vi "FITS read header.vi"() -> ()   [LabVIEW 2020]
panel:
  out "error out":errorcluster
  in  "error in":errorcluster
  out "Header":string[](array[string])
  out "data":string
  in  "Path":path
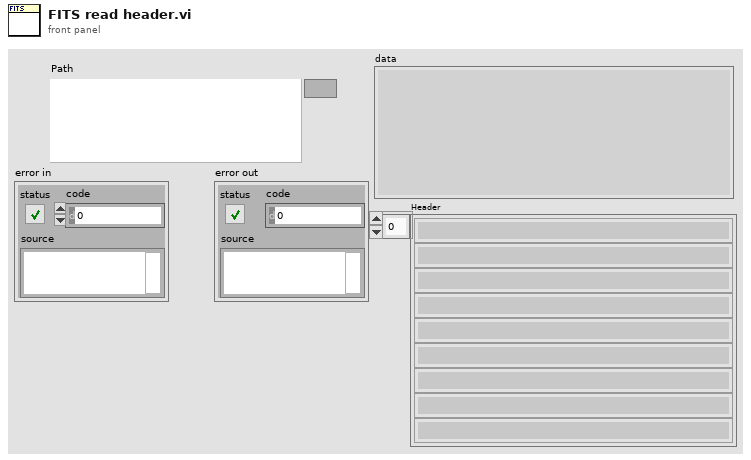
[diagram p1: front panel]
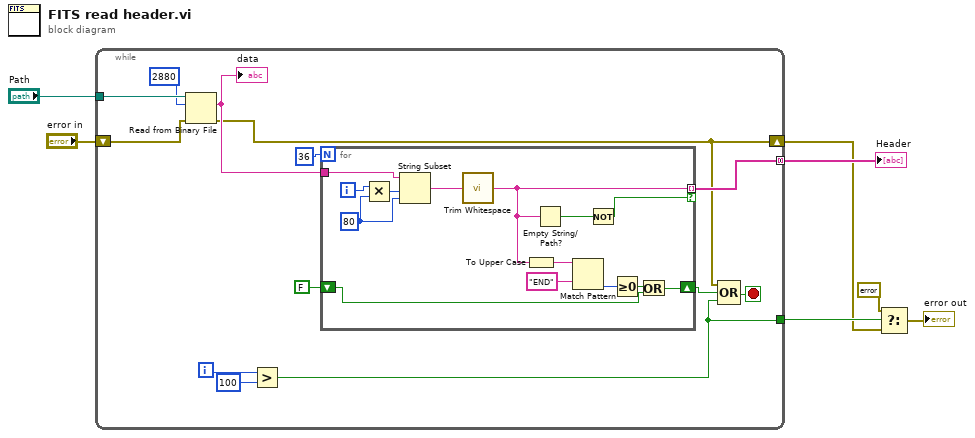
[diagram p0: block diagram]
diagram:
  n1 = while {
    tunnel: "Path" -> [w20]
    tunnel: [w16] -> w6 mode=concatenating
    tunnel: [w10] -> w4
    shift-right: [w8] -> w3
    shift-left: "error in" -> [w9]
    i -> [w13]
    stop <- w11 stop-if-true
    n2 = Read from Binary File(8:w9, 10:2880 ("count (1)"), 11:w20) -> (0:w8:errorcluster, 2:w18:string)  [unwired: 3 in, 2 out]
    "data" <- w18
    n3 = Greater?(x=w13, y=100) -> (0:w10:bool)
    n4 = for {
      N: 36 -> [_]
      tunnel: w18 -> [w34]
      tunnel: [w27] -> w16 mode=indexing if=w28
      shift-right: [w22] -> w14
      shift-left: FALSE -> [w21]
      i -> [w32]
      w31 = 80 ("length (rest)")
      n5 = Multiply(x=w32, y=w31) -> (x*y=w33:i32)
      n6 = String Subset(string=w34, offset (0)=w33, length (rest)=w31) -> (substring=w30:string)
      n7 = call <vilib>:"Trim Whitespace.vi"("string"=w30) -> ("trimmed string"=w27:string)  [unwired: 1 in]
      n8 = To Upper Case(1:w27) -> (0:w26:string)
      n9 = Empty String/Path?(string/path=w27) -> (empty?=w29:bool)
      n10 = Match Pattern(string=w26, regular expression="END") -> (offset past match=w24:i32)  [unwired: 1 in, 3 out]
      n11 = Not(x=w29) -> (.not. x?=w28:bool)
      n12 = Greater Or Equal To 0?(x=w24) -> (x >= 0?=w23:bool)
      n13 = Or(x=w23, y=w21) -> (x .or. y?=w22:bool)
    }
    n14 = Compound Arithmetic op=OR(w8, w14, w10) -> (w11:bool)
  }
  "Header" <- w6
  n15 = Select(t=errorcluster {"status"=TRUE, "code"=0, "source"="END keyword not found in header"}, s=w4, f=w3) -> (s? t:f=→"error out":errorcluster)
